vi "Plotter_Update_Receive_List_Values.vi"(8 "error in (no error)":errorcluster, 11 "Globals":T1) -> ()   [LabVIEW 2017]
uses:
  Controls/Plotter_Globals.ctl
  Classes/ADCP.lvclass
  Controls/Plotter_Queues.ctl
  Controls/Plotter_Queue_Command_and_Data.ctl
  Controls/Plotter_Commands.ctl
  Controls/Plotter_Plot_Parameter_and_Timestamp.ctl
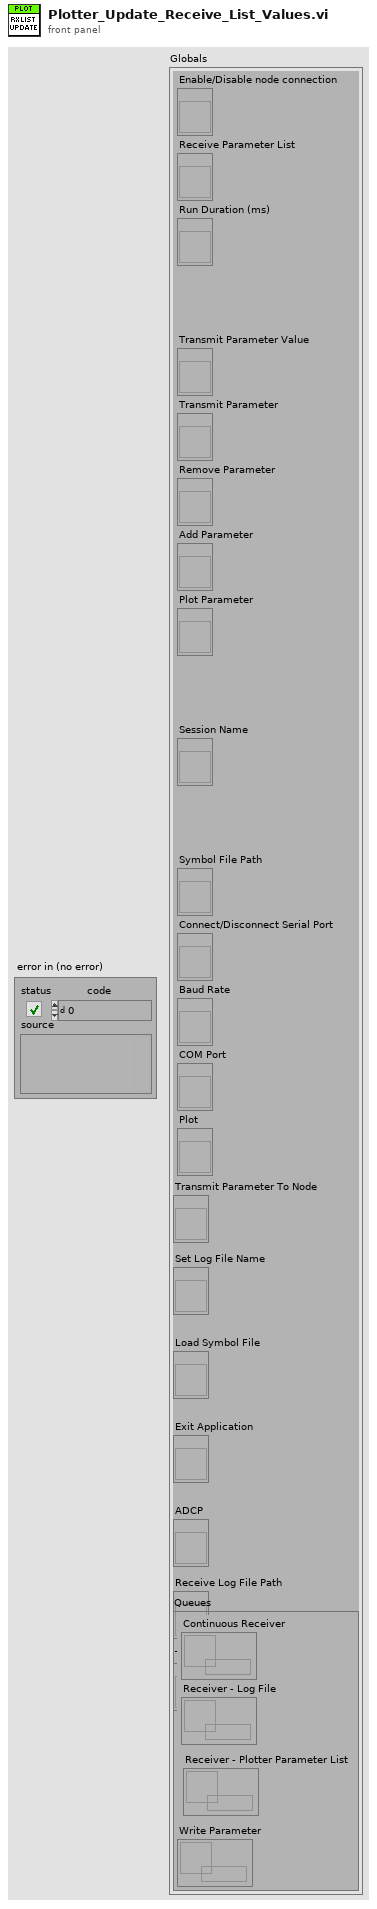
[diagram p1: front panel]
types:
  T1 = typedef "Plotter_Globals.ctl" = cluster{"Enable/Disable node connection":refnum<vi>, "Receive Parameter List":refnum<vi>, "Run Duration (ms)":refnum<vi>, "Transmit Parameter Value":refnum<vi>, "Transmit Parameter":refnum<vi>, "Remove Parameter":refnum<vi>, "Add Parameter":refnum<vi>, "Plot Parameter":refnum<vi>, "Session Name":refnum<vi>, "Symbol File Path":refnum<vi>, "Connect/Disconnect Serial Port":refnum<vi>, "Baud Rate":refnum<vi>, "COM Port":refnum<vi>, "Plot":refnum<vi>, "Transmit Parameter To Node":refnum<vi>, "Set Log File Name":refnum<vi>, "Load Symbol File":refnum<vi>, "Exit Application":refnum<vi>, "ADCP":refnum<vi>, "Transmit Log File Path":refnum<vi>, "Receive Log File Path":refnum<vi>, "Queues":T2}
  T2 = typedef "Plotter_Queues.ctl" = cluster{"Continuous Receiver":refnum<queue>, "Receiver - Log File":refnum<queue>, "Receiver - Plotter Parameter List":refnum<queue>, "Write Parameter":refnum<queue>}
  T3 = typedef "Plotter_Plot_Parameter_and_Timestamp.ctl" = cluster{"Parameter":string, "Value":string, "Time (ms)":u32}
  T4 = typedef "Plotter_Commands.ctl" = enum16{"Idle", "Cont_RX_Open_Node", "Cont_RX_Flush_Serial_Port", "Cont_Rx_Log_Write", "Plot_Update", "Exit"}
  T5 = typedef "Plotter_Queue_Command_and_Data.ctl" = cluster{"Commands":T4, "Data":variant}
  T6 = typedef "Plotter_Parameter_List_Record.ctl" = cluster{"Parameter":string, "Value":string}
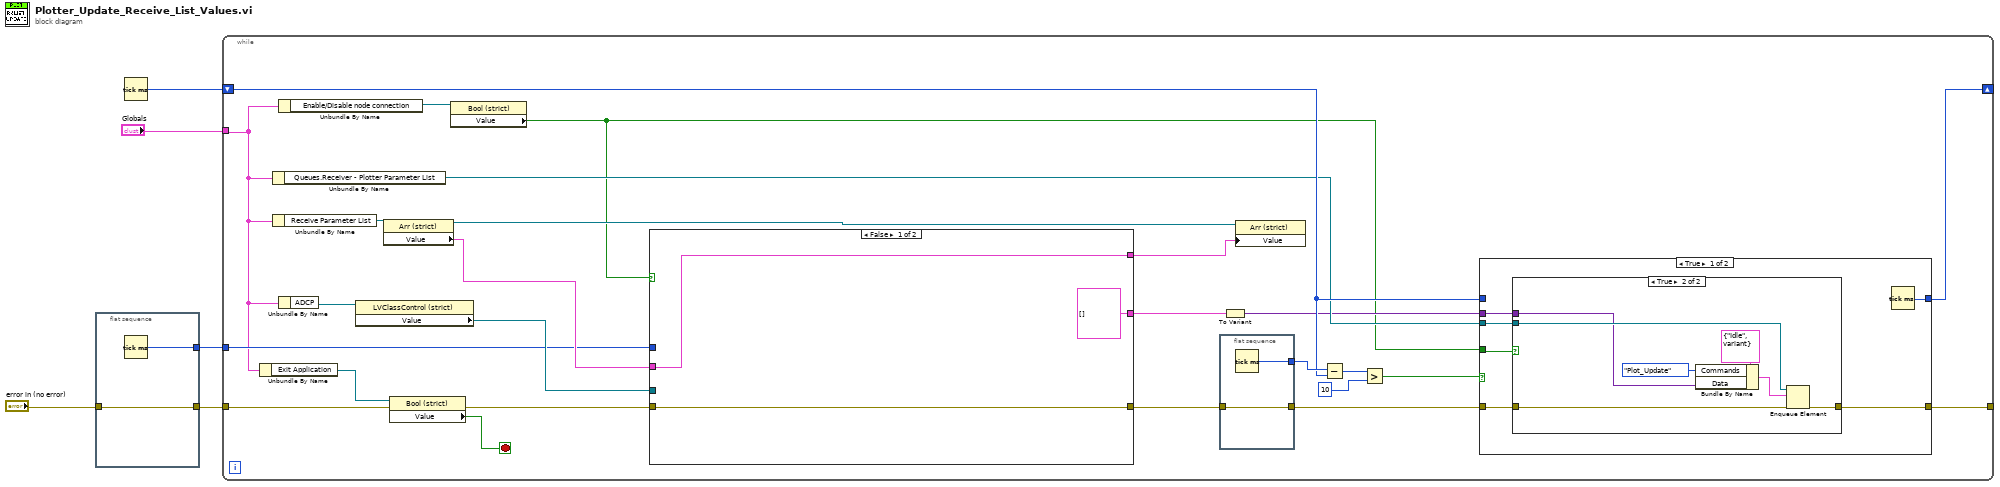
[diagram p0: block diagram]
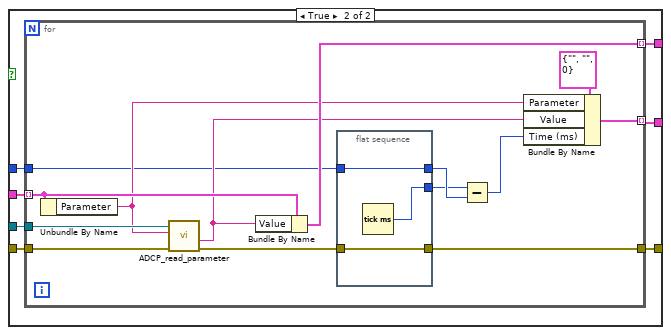
[diagram p2: hidden frame]
diagram:
  n1 = flat-sequence {
    tunnel: "error in (no error)" -> [w7]
    tunnel: [w7] -> w3
    tunnel: [w6] -> w2
    frame #0 {
      n2 = Tick Count (ms)() -> (millisecond timer value=w6:u32)
    }
  }
  n3 = Tick Count (ms)() -> (millisecond timer value=w1:u32)
  n4 = while {
    tunnel: "Globals" -> [w10]
    tunnel: w3 -> [w33]
    tunnel: w2 -> [w23]
    shift-right: [w16] -> _
    shift-left: w1 -> [w17]
    tunnel: [w11] -> _
    stop <- w31 stop-if-true
    n5 = Unbundle By Name(w10) -> ("Exit Application"=w32:refnum<vi>)
    n6 = Unbundle By Name(w10) -> ("Queues.Receiver - Plotter Parameter List"=w14:refnum<queue>)
    n7 = Unbundle By Name(w10) -> ("Receive Parameter List"=w27:refnum<vi>)
    n8 = Unbundle By Name(w10) -> ("Enable/Disable node connection"=w9:refnum<vi>)
    n9 = Unbundle By Name(w10) -> ("ADCP"=w30:refnum<vi>)
    n10 = property class="LVClassControl (strict)"(reference=w30) -> ("Value"=w28:refnum<class "ADCP.lvclass">)  [unwired: 1 in, 2 out]
    n11 = property class="Arr (strict)"(reference=w27) -> (reference out=w25:refnum<vi>, "Value"=w26:T6[])  [unwired: 1 in, 1 out]
    n12 = property class="Bool (strict)"(reference=w32, error in=w33) -> (error out=w29:errorcluster, "Value"=w31:bool)  [unwired: 1 out]
    n13 = property class="Bool (strict)"(reference=w9) -> ("Value"=w8:bool)  [unwired: 1 in, 2 out]
    n14 = case shown="False" w8 {
      tunnel: w29 -> [w36 w43]
      tunnel: w28 -> [_ w42]
      tunnel: w26 -> [w35 w41]
      tunnel: [w35 w40] -> w24
      tunnel: w23 -> [_ w39]
      tunnel: [T3[] [] w38] -> w22
      tunnel: [w36 w37] -> w21
      frame False {
      }
      frame True {
        n15 = for {
          tunnel: w43 -> [w57]
          tunnel: w42 -> [w56]
          tunnel: w41 -> [w55] mode=indexing
          tunnel: [w54] -> w40 mode=indexing
          tunnel: w39 -> [w49]
          tunnel: [w45] -> w37
          tunnel: [w44] -> w38 mode=indexing
          n16 = Unbundle By Name(w55) -> ("Parameter"=w52:string)
          n17 = call "ADCP_read_parameter.vi"("error in (no error)"=w57, "Parameter Name"=w52, "ADCP In"=w56) -> ("error out"=w50:errorcluster, "Parameter Value"=w51:string)  [unwired: 5 in, 2 out]
          n18 = Bundle By Name(cluster=w55, "Value"=w51) -> (w54:T6)
          n19 = flat-sequence {
            tunnel: w50 -> [w60]
            tunnel: [w60] -> w45
            tunnel: w49 -> [w59]
            tunnel: [w59] -> w48
            tunnel: [w58] -> w47
            frame #0 {
              n20 = Tick Count (ms)() -> (millisecond timer value=w58:u32)
            }
          }
          n21 = Subtract(x=w47, y=w48) -> (x-y=w46:u32)
          n22 = Bundle By Name(cluster=T3 {"Parameter"="", "Value"="", "Time (ms)"=0}, "Parameter"=w52, "Value"=w51, "Time (ms)"=w46) -> (w44:T3)
        }
      }
    }
    n23 = flat-sequence {
      tunnel: w21 -> [w78]
      tunnel: [w78] -> w15
      tunnel: [w77] -> w20
      frame #0 {
        n24 = Tick Count (ms)() -> (millisecond timer value=w77:u32)
      }
    }
    n25 = To Variant(anything=w22) -> (Variant=w13:variant)
    n26 = property class="Arr (strict)"(reference=w25, "Value"=w24) -> ()  [unwired: 1 in, 2 out]
    n27 = Subtract(x=w20, y=w17) -> (x-y=w12:u32)
    n28 = Greater?(x=w12, y=u32 10) -> (0:w18:bool)
    n29 = case shown="True" w18 {
      tunnel: w17 -> [_ w76]
      tunnel: [w66 w76] -> w16
      tunnel: w15 -> [w65 w75]
      tunnel: [w62 w75] -> w11
      tunnel: w14 -> [w64 _]
      tunnel: w13 -> [w63 _]
      tunnel: w8 -> [w61 _]
      frame True {
        n30 = case shown="True" w61 {
          tunnel: w65 -> [w67 w74]
          tunnel: w64 -> [_ w72]
          tunnel: w63 -> [_ w69]
          tunnel: [w67 w73] -> w62
          frame False {
          }
          frame True {
            n31 = Bundle By Name(cluster=T5 {"Commands"=enum."Idle", "Data"=variant} ("Plotter_Queue_Command_and_Data"), "Commands"=Plotter_Commands."Plot_Update", "Data"=w69) -> (w68:T5)
            n32 = Enqueue Element(queue=w72, element=w68, error in (no error)=w74) -> (error out=w73:errorcluster)  [unwired: 1 in, 2 out]
          }
        }
        n33 = Tick Count (ms)() -> (millisecond timer value=w66:u32)
      }
      frame False {
      }
    }
  }
